vi "Heater_Setpoint_Panel.vi"() -> ()   [LabVIEW 2010]
uses:
  Heater_Setpoint.ctl
  ADAM Controls/Channel_names.ctl
  ADAM Controls/Channel_State.ctl
panel:
  in  "Mode":u16(ring) items=["Only Show Setpoints Above Zero", "Show all Setpoints"]
  in  "Setpoints Out":T1[](array[typedef])
  out "Messages":string
  in  "OK":bool
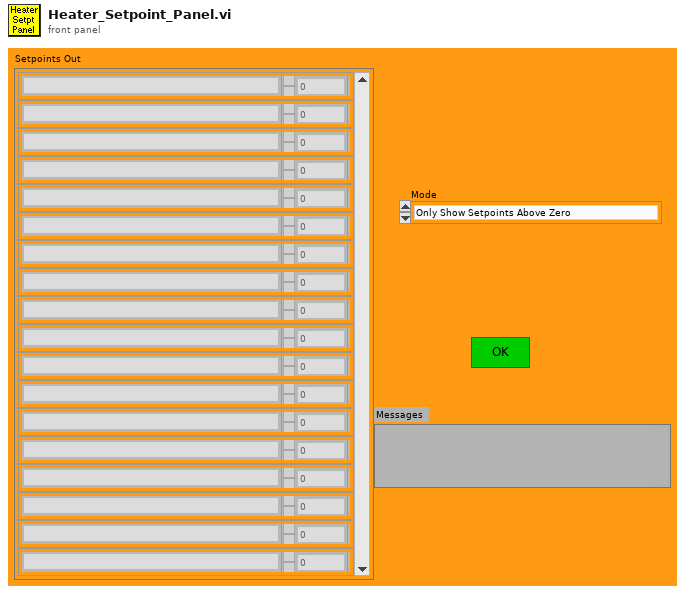
[diagram p1: front panel]
types:
  T1 = typedef "Heater_Setpoint.ctl" = cluster{"Ch Name":string, "Setpoint":dbl}
  T2 = typedef "Channel_names.ctl" = enum16{"Active Only", "Active + Off", "All Channels"}
  T3 = typedef "Channel_State.ctl" = enum16{"On", "Off", "Always On", "Always Off"}
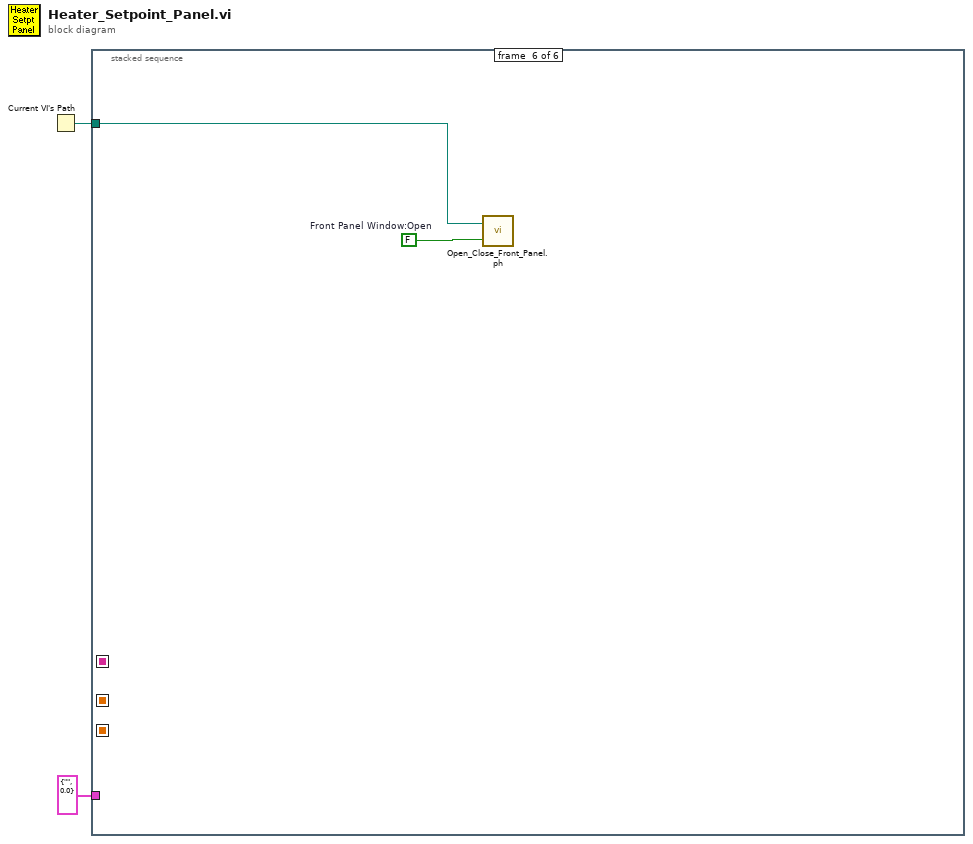
[diagram p0: block diagram]
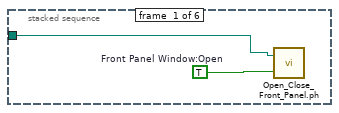
[diagram p2: hidden frame]
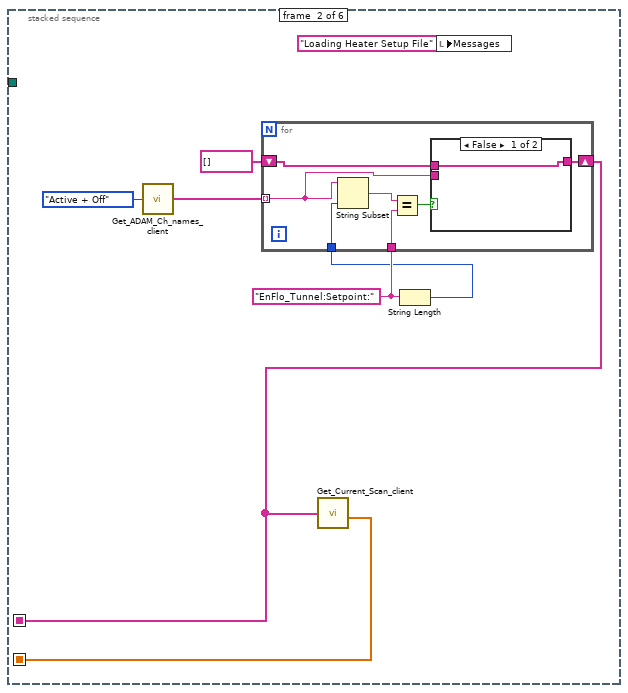
[diagram p3: hidden frame]
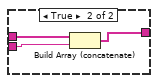
[diagram p4: hidden frame]
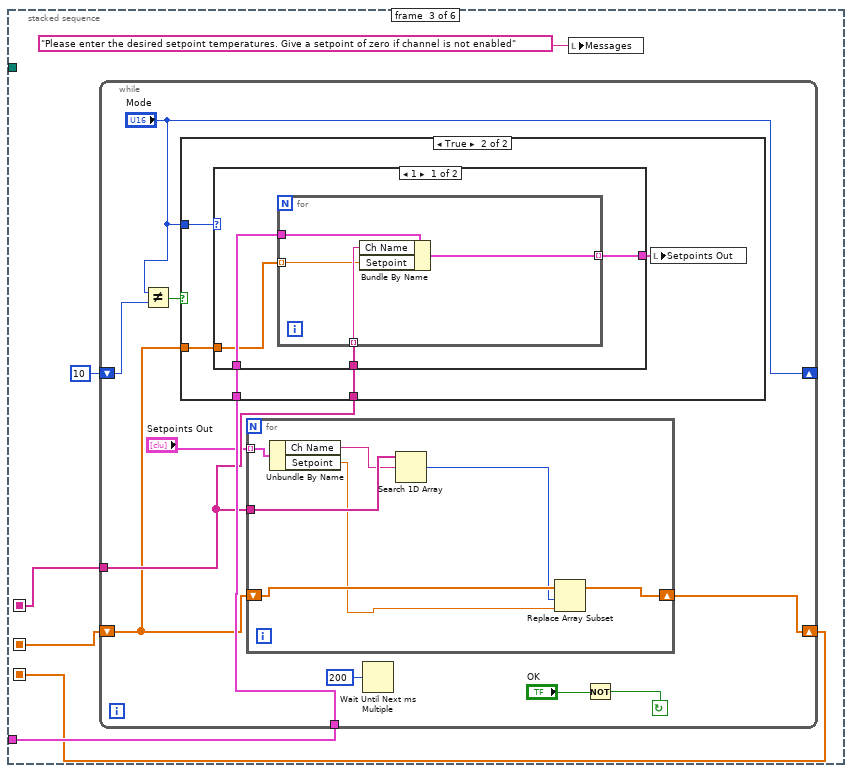
[diagram p5: hidden frame]
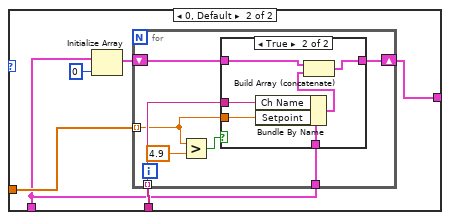
[diagram p7: hidden frame]
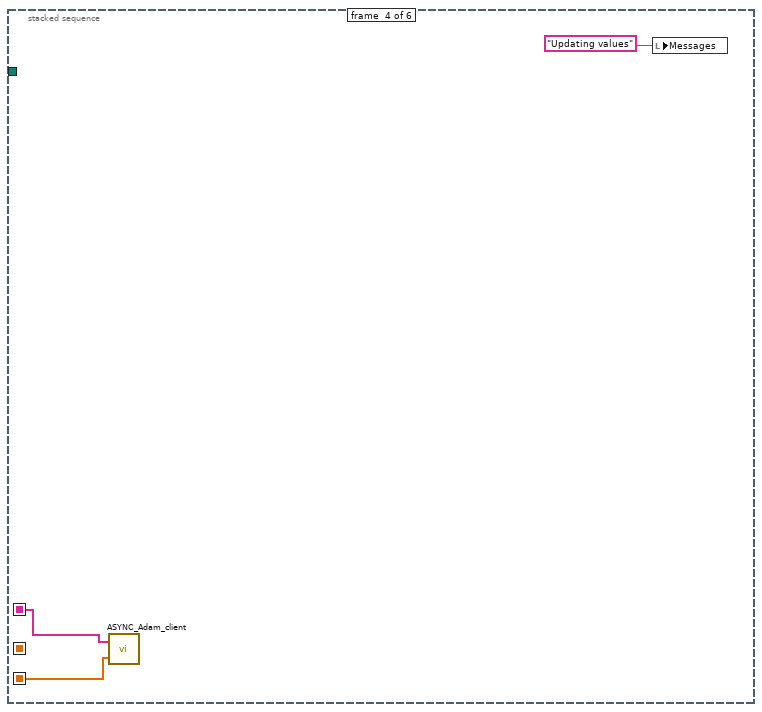
[diagram p9: hidden frame]
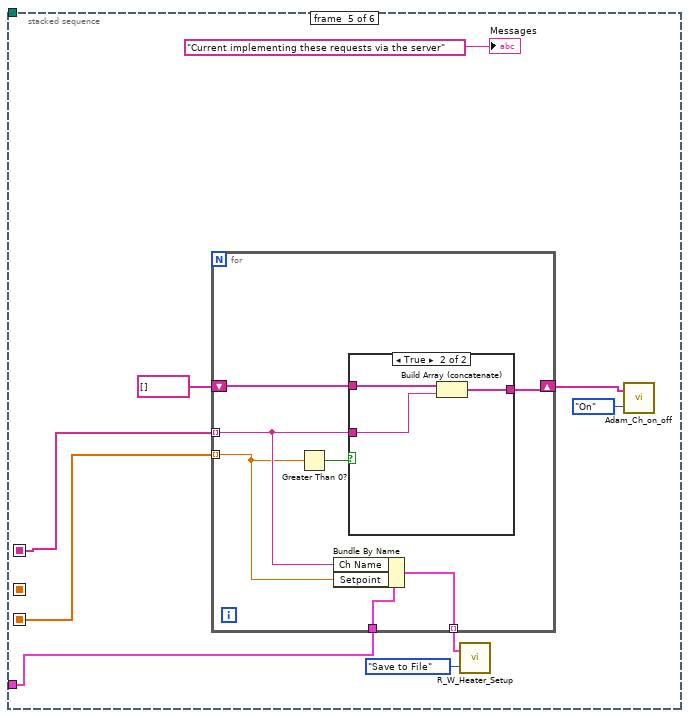
[diagram p10: hidden frame]
diagram:
  n1 = Current VI's Path() -> (path=w2:path)
  n2 = stacked-sequence {
    seq-local: [_ w5 _ _ _ _] -> [_ _ w26 _ _ _]
    seq-local: [_ w6 _ _ _ _] -> [_ _ w28 w82 w87 _]
    seq-local: [_ _ w24 _ _ _] -> [_ _ _ w81 w86 _]
    tunnel: w2 -> [w4 _ _ _ _ w104]
    tunnel: T1 {"Ch Name"="", "Setpoint"=0.0} ("Cluster") -> [_ _ w27 _ w85 _]
    frame #0 {
      w3 = TRUE  # Front Panel Window:Open
      n3 = call "Open_Close_Front_Panel.ph.vi"("Front Panel Window:Open"=w3, "VI path"=w4) -> ()  [unwired: 2 out]
    }
    frame #1 {
      w10 = "EnFlo_Tunnel:Setpoint:"
      n4 = call "Get_ADAM_Ch_names_client.vi"("Channel names set"=Channel_names."Active + Off") -> ("Ch names"=w7:string[])
      n5 = String Length(string=w10) -> (length=w9:i32)
      n6 = for {
        shift-right: [w13] -> w6
        shift-left: string[] [] -> [w15]
        tunnel: w7 -> [w14] mode=indexing
        tunnel: w9 -> [w19]
        tunnel: w10 -> [w18]
        n7 = String Subset(string=w14, length (rest)=w19) -> (substring=w17:string)  [unwired: 1 out]
        n8 = Equal?(x=w17, y=w18) -> (x = y?=w16:bool)
        n9 = case shown="False" w16 {
          tunnel: w15 -> [w20 w23]
          tunnel: w14 -> [_ w22]
          tunnel: [w20 w21] -> w13
          frame False {
          }
          frame True {
            n10 = Build Array (concatenate)(w23, w22) -> (w21:string[])
          }
        }
      }
      n11 = call "Get_Current_Scan_client.vi"("ADAM Ch Names"=w6) -> ("Numerical Values"=w5:dbl[])  [unwired: 3 out]
      n12 = local write "Messages"("Loading Heater Setup File" ("Messages")) -> ()
    }
    frame #2 {
      n13 = while {
        tunnel: w28 -> [w32]
        tunnel: w27 -> [w33]
        shift-right: [w37] -> w24
        shift-left: w26 -> [w31]
        shift-right: ["Mode"] -> _
        shift-left: u16 10 ("Mode") -> [w36]
        stop <- w39 continue-if-true
        n14 = Not Equal?(x="Mode", y=w36) -> (x != y?=w35:bool)
        n15 = case shown="True" w35 {
          tunnel: "Mode" -> [_ w45]
          tunnel: w33 -> [_ w44]
          tunnel: w32 -> [_ w43]
          tunnel: w31 -> [_ w42]
          frame False {
          }
          frame True {
            n16 = case shown="1" w45 {
              tunnel: w44 -> [w49 w56]
              tunnel: w43 -> [w48 w58]
              tunnel: w42 -> [w47 w59]
              tunnel: [w46 w57] -> w41
              frame 1 {
                n17 = for {
                  tunnel: w49 -> [w53]
                  tunnel: w48 -> [w52] mode=indexing
                  tunnel: w47 -> [w51] mode=indexing
                  tunnel: [w50] -> w46 mode=indexing
                  n18 = Bundle By Name(cluster=w53, "Ch Name"=w52, "Setpoint"=w51) -> (w50:T1)
                }
              }
              frame 0, Default {
                n19 = Initialize Array(w56, 0 ("dimension size")) -> (w54:T1[])
                n20 = for {
                  tunnel: w58 -> [w66] mode=indexing
                  tunnel: w59 -> [w65] mode=indexing
                  tunnel: w56 -> [w62]
                  shift-right: [w61] -> w57
                  shift-left: w54 -> [w60]
                  n21 = Greater?(x=w65, y=4.9) -> (0:w63:bool)
                  n22 = case shown="True" w63 {
                    tunnel: w66 -> [_ w73]
                    tunnel: w65 -> [_ w72]
                    tunnel: w62 -> [_ w71]
                    tunnel: [w67 w69] -> w61
                    tunnel: w60 -> [w67 w68]
                    frame False {
                    }
                    frame True {
                      n23 = Bundle By Name(cluster=w71, "Ch Name"=w73, "Setpoint"=w72) -> (w70:T1)
                      n24 = Build Array (concatenate)(w68, w70) -> (w69:T1[])
                    }
                  }
                }
              }
            }
            n25 = local write "Setpoints Out"(w41) -> ()
          }
        }
        n26 = for {
          tunnel: "Setpoints Out" -> [w80] mode=indexing
          tunnel: w32 -> [w79]
          shift-right: [w76] -> w37
          shift-left: w31 -> [w77]
          n27 = Unbundle By Name(w80) -> ("Ch Name"=w78:string, "Setpoint"=w74:dbl)
          n28 = Search 1D Array(1D array=w79, element=w78) -> (index of element=w75:i32)  [unwired: 1 out]
          n29 = Replace Array Subset(array=w77, new element=w74, index=w75) -> (w76:dbl[])
        }
        n30 = Wait Until Next ms Multiple(millisecond multiple=u32 200) -> ()  [unwired: 1 out]
        n31 = Not(x="OK") -> (.not. x?=w39:bool)
      }
      n32 = local write "Messages"("Please enter the desired setpoint temperatures. Give a setpoint of zero if channel is not enabled" ("Messages")) -> ()
    }
    frame #3 {
      n33 = call "ASYNC_Adam_client.vi"("Values"=w81, "Channel Names"=w82) -> ()  [unwired: 2 out]
      n34 = local write "Messages"("Updating values" ("Messages")) -> ()
    }
    frame #4 {
      n35 = for {
        shift-right: [w98] -> w88
        shift-left: string[] [] -> [w99]
        tunnel: w87 -> [w96] mode=indexing
        tunnel: w86 -> [w93] mode=indexing
        tunnel: w85 -> [w97]
        tunnel: [w95] -> w84 mode=indexing
        n36 = Greater Than 0?(x=w93) -> (x > 0?=w94:bool)
        n37 = Bundle By Name(cluster=w97, "Ch Name"=w96, "Setpoint"=w93) -> (w95:T1)
        n38 = case shown="True" w94 {
          tunnel: w99 -> [w100 w103]
          tunnel: w96 -> [_ w102]
          tunnel: [w100 w101] -> w98
          frame False {
          }
          frame True {
            n39 = Build Array (concatenate)(w103, w102) -> (w101:string[])
          }
        }
      }
      n40 = call "R_W_Heater_Setup.vi"("Mode"=enum16{"Load from File", "Save to File"}."Save to File", "Setpoints In"=w84) -> ()  [unwired: 2 out]
      n41 = call "Adam_Ch_on_off.vi"("Ch State"=Channel_State."On", "ADAM Ch Names"=w88) -> ()  [unwired: 1 out]
      "Messages" <- "Current implementing these requests via the server" ("Messages")
    }
    frame #5 {
      w105 = FALSE  # Front Panel Window:Open
      n42 = call "Open_Close_Front_Panel.ph.vi"("Front Panel Window:Open"=w105, "VI path"=w104) -> ()  [unwired: 2 out]
    }
  }
